vi "confirm_measured_values_DFA.vi"(10 "LIDAR raw data":u8) -> (1 "new_measurement?":bool, 2 "last measured value":u16)   [LabVIEW 2009]
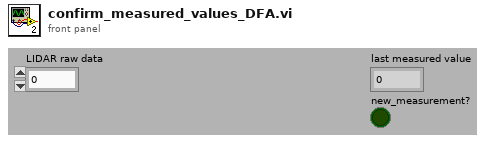
[diagram p1: front panel]
types:
  T1 = enum16{"confirm check sum", "check status byte", "read measured values", "confirm measurement", "confirm command", "read message length", "read address", "wait for \"02\""}
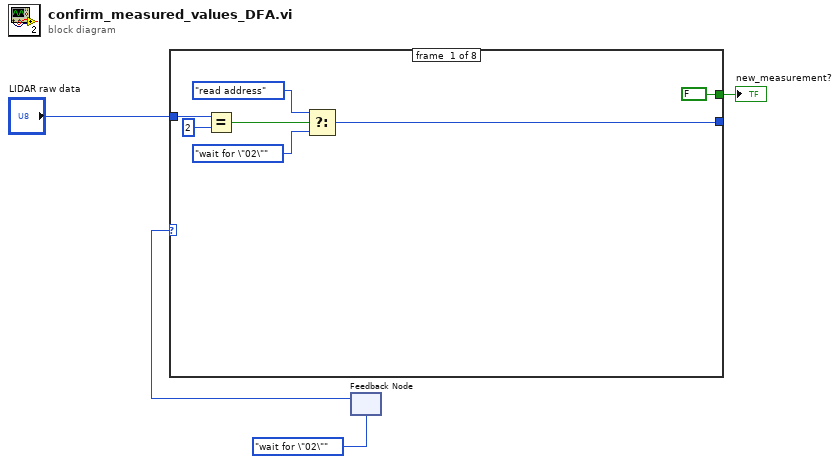
[diagram p0: block diagram]
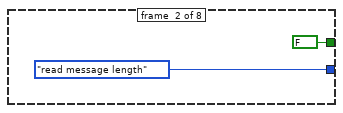
[diagram p2: hidden frame]
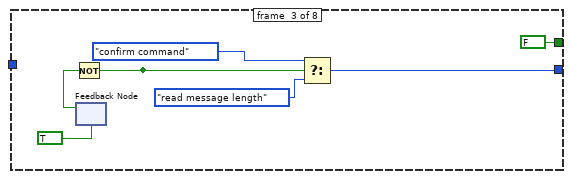
[diagram p3: hidden frame]
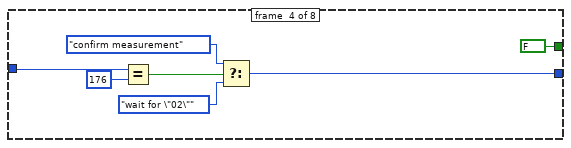
[diagram p4: hidden frame]
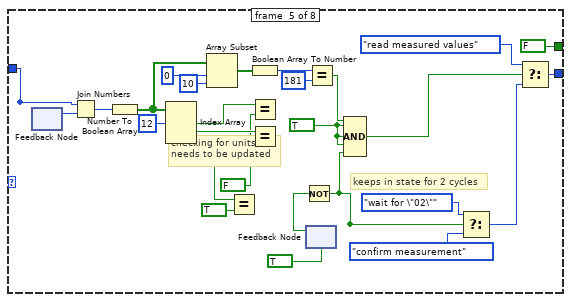
[diagram p5: hidden frame]
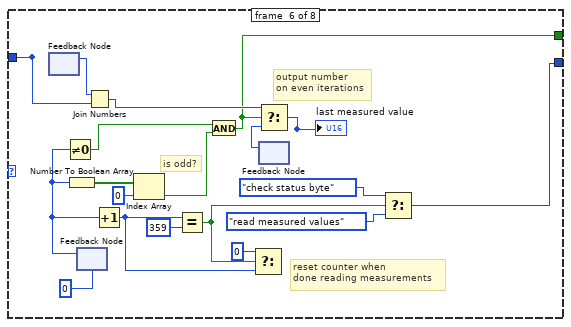
[diagram p6: hidden frame]
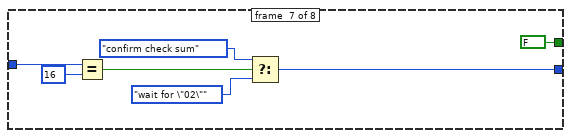
[diagram p7: hidden frame]
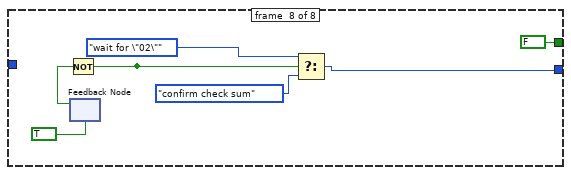
[diagram p8: hidden frame]
diagram:
  n1 = feedback #1(T1."wait for \"02\"") -> (w4:T1)
  n2 = case shown="\"read measured values\"" w4 {
    tunnel: "LIDAR raw data" -> [w12 _ _ w28 w31 w74 w82 _]
    tunnel: [w7 T1."read message length" w17 w23 w41 w58 w77 w84] -> w3
    tunnel: [FALSE FALSE FALSE FALSE FALSE w56 FALSE FALSE] -> w1
    frame #0 {
      n3 = Equal?(x=w12, y=i8 2) -> (x = y?=w10:bool)
      n4 = Select(t=T1."read address", s=w10, f=T1."wait for \"02\"") -> (s? t:f=w7:T1)
    }
    frame #1 {
    }
    frame #2 {
      n5 = feedback #2(TRUE) -> (w21:bool)
      n6 = Not(x=w21) -> (.not. x?=w19:bool)
      n7 = Select(t=T1."confirm command", s=w19, f=T1."read message length") -> (s? t:f=w17:T1)
    }
    frame #3 {
      n8 = Equal?(x=w28, y=u8 176) -> (x = y?=w26:bool)
      n9 = Select(t=T1."confirm measurement", s=w26, f=T1."wait for \"02\"") -> (s? t:f=w23:T1)
    }
    frame #4 {
      w30 = TRUE
      w50 = FALSE ("y")
      # "checking for units\nneeds to be updated"
      # "keeps in state for 2 cycles"
      n10 = feedback #3() -> (w32:u8)  [unwired: 1 in]
      n11 = Join Numbers(hi=w31, lo=w32) -> ((hi.lo)=w55:u16)
      n12 = Number To Boolean Array(number=w55) -> (Boolean array=w48:bool[])
      n13 = Index Array(array=w48, index #1=12 ("index")) -> (element #1=w49:bool, element #2=w51:bool, element #3=w53:bool)  [unwired: 2 in]
      n14 = Array Subset(array=w48, index=0, length=10) -> (w45:bool[])
      n15 = Equal?(x=w53, y=TRUE) -> ()  [unwired: 1 out]
      n16 = Boolean Array To Number(Boolean array=w45) -> (number=w44:u16)
      n17 = Equal?(x=w49, y=w50) -> ()  [unwired: 1 out]
      n18 = Equal?(x=w51, y=w50) -> ()  [unwired: 1 out]
      n19 = feedback #4(TRUE) -> (w39:bool)
      n20 = Not(x=w39) -> (.not. x?=w33:bool)
      n21 = Equal?(x=w44, y=u16 181) -> (x = y?=w42:bool)
      n22 = Compound Arithmetic op=AND(w42, w30, w30, w30, w33) -> (w35:bool)
      n23 = Select(t=T1."wait for \"02\"", s=w33, f=T1."confirm measurement") -> (s? t:f=w36:T1)
      n24 = Select(t=T1."read measured values", s=w35, f=w36) -> (s? t:f=w41:T1)
    }
    frame #5 {
      # "is odd?"
      # "output number\non even iterations"
      # "reset counter when\ndone reading measurements"
      n25 = feedback #5() -> (w75:u8)  [unwired: 1 in]
      n26 = feedback #6(i16 0) -> (w66:i16)
      n27 = Not Equal To 0?(x=w66) -> (x != 0?=w65:bool)
      n28 = Number To Boolean Array(number=w66) -> (Boolean array=w71:bool[])
      n29 = Join Numbers(hi=w75, lo=w74) -> ((hi.lo)=w69:u16)
      n30 = Increment(x=w66) -> (x+1=w63:i16)
      n31 = Index Array(array=w71, index=0) -> (element=w57:bool)
      n32 = Equal?(x=w63, y=i16 359) -> (x = y?=w61:bool)
      n33 = And(x=w65, y=w57) -> (x .and. y?=w56:bool)
      n34 = Select(t=i16 0, s=w61, f=w63) -> (s? t:f=w64:i16)
      n35 = feedback #7() -> (w67:u16)  [unwired: 1 in]
      n36 = Select(t=w69, s=w56, f=w67) -> (s? t:f=w68:u16)
      "last measured value" <- w68
      n37 = Select(t=T1."check status byte", s=w61, f=T1."read measured values") -> (s? t:f=w58:T1)
    }
    frame #6 {
      n38 = Equal?(x=w82, y=u8 16) -> (x = y?=w80:bool)
      n39 = Select(t=T1."confirm check sum", s=w80, f=T1."wait for \"02\"") -> (s? t:f=w77:T1)
    }
    frame #7 {
      n40 = feedback #8(TRUE) -> (w89:bool)
      n41 = Not(x=w89) -> (.not. x?=w87:bool)
      n42 = Select(t=T1."wait for \"02\"", s=w87, f=T1."confirm check sum") -> (s? t:f=w84:T1)
    }
  }
  "new_measurement?" <- w1
